vi "T7 Stream Read KAG-v2.vi"(0 "Connection ID In":refnum<k5>, 7 "Stream Configuration":T2={"Scan Rate (Hz)"=1000.0, "Samples Per Packet"=512, "Resolution Index"=0, "Buffer Size (bytes)"=32768, "NumScans"=1500, "Read Timeout (ms)"=5000, "Scan Table"=[{"Channel"=0, "BipGain"=0, "Input Config"="Single-Ended"}, {"Channel"=1, "BipGain"=0, "Input Config"="Single-Ended"}, {"Channel"=2, "BipGain"=0, "Input Config"="Single-Ended"}, {"Channel"=3, "BipGain"=0, "Input Config"="Single-Ended"}]} {"Samples Per Packet" max=512 step=1; "Buffer Size (bytes)" max=32768 step=1; "Resolution Index" max=8 step=1; "Scan Rate (Hz)" max=100000; "Scan Table"."BipGain" items=["x1", "x10", "x100", "x1000"]; "Scan Table"."Channel" step=1}, 9 "Secondary Stream Configurations":T1={"Settling Delay (*5 us)"=0.0, "Clock Source"=0, "Auto Target"=1} {"Auto Target" max=255 step=1; "Clock Source" max=2 step=2; "Settling Delay (*5 us)" min=0 max=5000 step=1}, 11 "error in":errorcluster) -> (6 "Read Array":u8[](array[numeric]) format="%.0x", 8 "TCP Data":string, 15 "error out":errorcluster)   [LabVIEW 2022 SP3]
doc: "Read Stream Data at Ethernet Socket 702."
uses:
  T7 Stream Config KAG.ctl
  T7 Secondary Configs KAG.ctl
  T7 Stream Globals KAG.vi
panel:
  in  "Tab Control":enum32{"TCP Read Data"}(tab)
  out "# of bytes received":i32
  out "# Bytes to Read":i32
  out "Scan Interval(s)":dbl
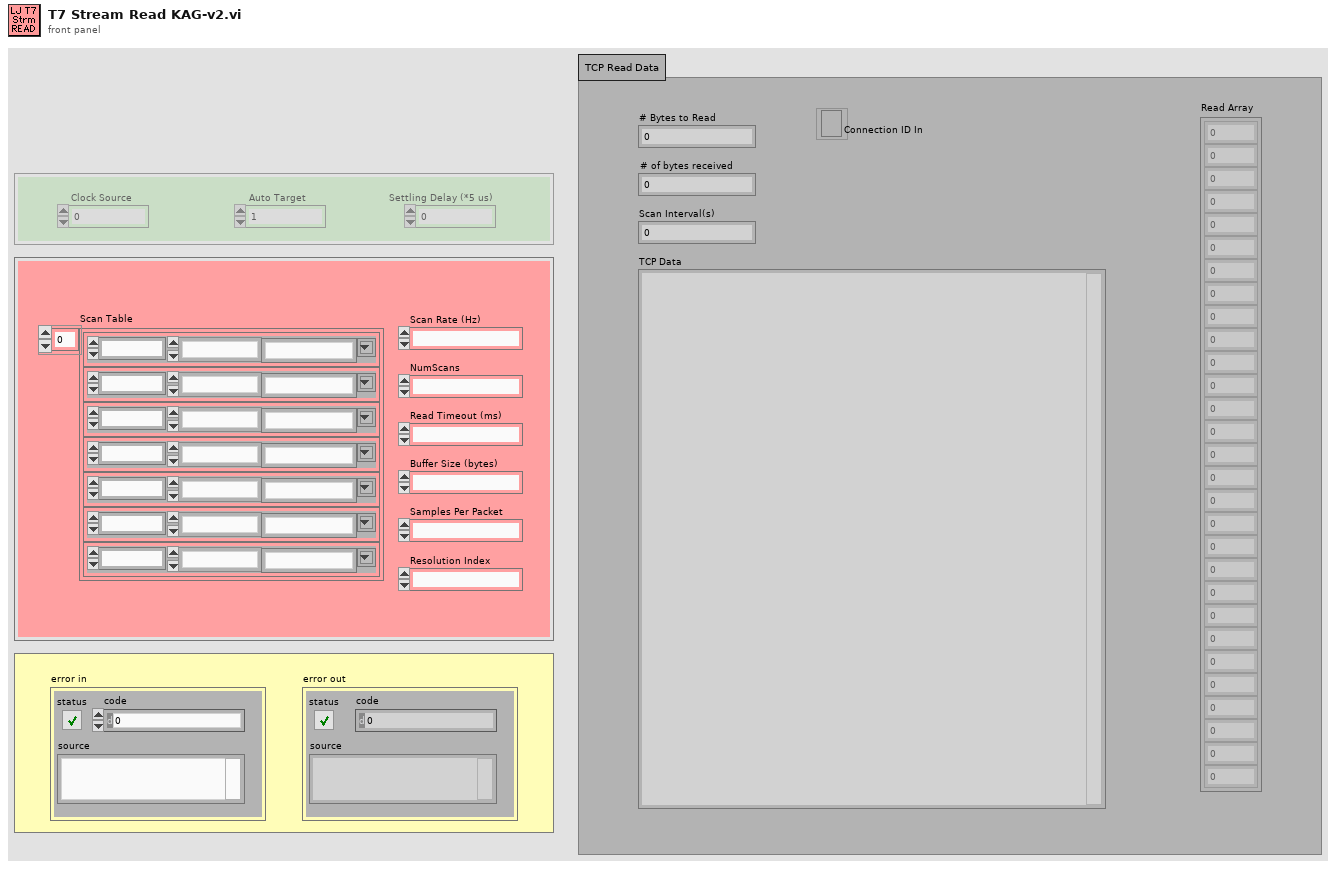
[diagram p1: front panel]
types:
  T1 = typedef "T7 Secondary Configs KAG.ctl" = cluster{"Settling Delay (*5 us)":sgl, "Clock Source":u32, "Auto Target":u32}
  T2 = typedef "T7 Stream Config KAG.ctl" = cluster{"Scan Rate (Hz)":sgl, "Samples Per Packet":u32, "Resolution Index":u32, "Buffer Size (bytes)":u32, "NumScans":u32, "Read Timeout (ms)":u32, "Scan Table":cluster{"Channel":u32, "BipGain":u32, "Input Config":string}[]}
  T3 = cluster{"Channel":u32, "BipGain":u32, "Input Config":string}[]
  T4 = typedef "T7 IP Config KAG.ctl" = cluster{"Connection ID In":refnum<k5>, "Connection ID Out":refnum<k5>, "Device IP":string, "Port":i32}
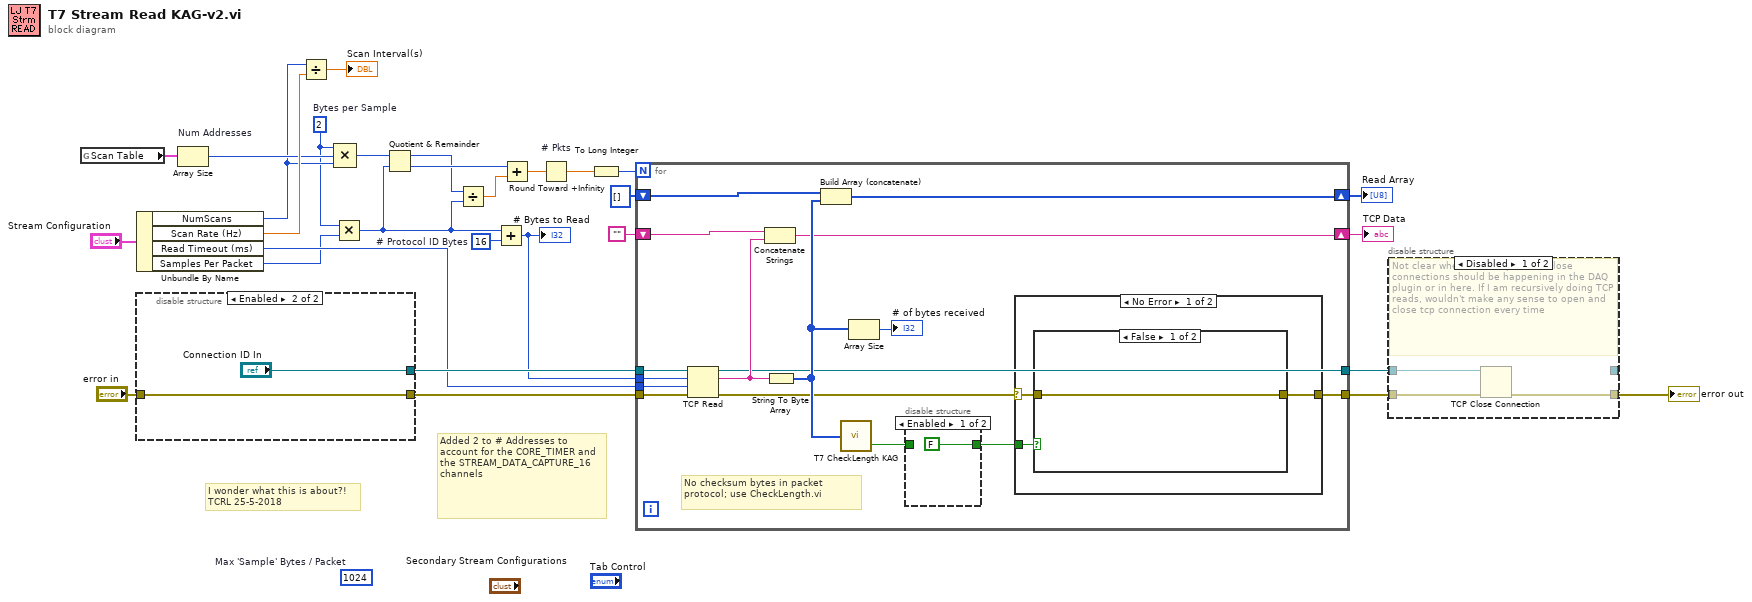
[diagram p0: block diagram]
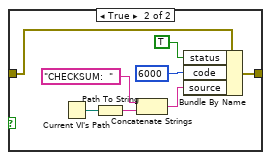
[diagram p4: hidden frame]
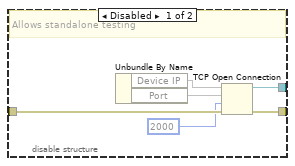
[diagram p6: hidden frame]
diagram:
  w2 = u32 16  # # Protocol ID Bytes
  (unwired) 1024  # Max 'Sample' Bytes / Packet
  w8 = 2  # Bytes per Sample
  # "I wonder what this is about?!\nTCRL 25-5-2018"
  # "Added 2 to # Addresses to account for the CORE_TIMER and the STREAM_DATA_CAPTURE_16 channels"
  n1 = global read "T7 Stream Globals KAG.vi" "Scan Table"() -> (w23:T3)
  n2 = Unbundle By Name("Stream Configuration") -> ("NumScans"=w18:u32, "Scan Rate (Hz)"=w20:sgl, "Read Timeout (ms)"=w21:u32, "Samples Per Packet"=w9:u32)
  n3 = disable-structure shown="Enabled" {
    disable-tunnel: "error in" -> [w36 w38]
    disable-tunnel: [w35 w38] -> w27
    disable-tunnel: [w34 "Connection ID In"] -> w26
    frame Disabled {
      # "Allows standalone testing"
      n4 = Unbundle By Name() -> (w33:T4, "Device IP"=w32, "Port"=w31)
      n5 = TCP Open Connection(address=w32, remote port or service name=w31, timeout ms (60000)=2000, error in (no error)=w36) -> (connection ID=w34:refnum<k5>, error out=w35:errorcluster)  [unwired: 1 out]
    }
    frame Enabled {
    }
  }
  n6 = Array Size "Num Addresses"(array=w23) -> (size(s)=w19:i32)
  n7 = Divide(x=w18, y=w20) -> (x/y=→"Scan Interval(s)":sgl)
  n8 = Compound Arithmetic op=MULTIPLY(w8, w19, w18) -> (w17:u32)
  n9 = Multiply(x=w8, y=w9) -> (x*y=w7:u32)
  n10 = Quotient & Remainder(x=w17, y=w7) -> (x-y*floor(x/y)=w6:u32, floor(x/y)=w15:u32)
  n11 = Divide(x=w6, y=w7) -> (x/y=w16:dbl)
  n12 = Add(x=w7, y=w2) -> (x+y=w1:u32)
  "# Bytes to Read" <- w1
  n13 = Add(x=w15, y=w16) -> (x+y=w14:dbl)
  n14 = Round Toward +Infinity "# Pkts"(x=w14) -> (ceil(x): smallest int >= x=w13:dbl)
  n15 = To Long Integer(number=w13) -> (32bit integer=w12:i32)
  n16 = for {
    N: w12 -> [_]
    tunnel: w27 -> [w53]
    tunnel: w26 -> [w52]
    tunnel: w21 -> [w49]
    shift-right: [w47] -> w25
    shift-left: u8[] [] ("unsigned byte array") -> [w46]
    shift-right: [w43] -> w29
    shift-left: "" -> [w45]
    tunnel: [w42] -> w4
    tunnel: [w41] -> w5
    tunnel: w1 -> [w39]
    # "No checksum bytes in packet protocol; use CheckLength.vi"
    n17 = TCP Read(connection ID=w52, bytes to read=w39, error in (no error)=w53, 9:w49) -> (connection ID out=w41:refnum<k5>, data out=w44:string, error out=w40:errorcluster)  [unwired: 1 out]
    n18 = Concatenate Strings(w45, w44) -> (w43:string)
    n19 = String To Byte Array(string=w44) -> (unsigned byte array=w48:u8[])
    n20 = Build Array (concatenate)(w46, w48) -> (w47:u8[])
    n21 = call "T7 CheckLength KAG.vi"("Array"=w48) -> ("CheckLength Error"=w50:bool)  [unwired: 1 out]
    n22 = Array Size(array=w48) -> (size(s)=→"# of bytes received":i32)
    n23 = disable-structure shown="Enabled" {
      disable-tunnel: [FALSE w56] -> w51
      disable-tunnel: w50 -> [_ w56]
      frame Enabled {
      }
      frame Disabled {
      }
    }
    n24 = case shown="No Error" w40 {
      selector: w40 -> [w59 w69]
      tunnel: [w58 w69] -> w42
      tunnel: w51 -> [w57 _]
      frame No Error {
        n25 = case shown="False" w57 {
          tunnel: w59 -> [w60 w68]
          tunnel: [w60 w67] -> w58
          frame False {
          }
          frame True {
            n26 = Current VI's Path() -> (path=w65:path)
            n27 = Path To String(path=w65) -> (string=w63:string)
            n28 = Concatenate Strings("CHECKSUM:  " ("Substring"), w63) -> (w62:string)
            n29 = Bundle By Name(cluster=w68, "status"=TRUE, "code"=u32 6000 ("y"), "source"=w62) -> (w67:errorcluster)
          }
        }
      }
      frame Error {
      }
    }
  }
  "Read Array" <- w25
  "TCP Data" <- w29
  n30 = disable-structure shown="Disabled" {
    disable-tunnel: w5 -> [w72 w74]
    disable-tunnel: w4 -> [w71 w73]
    disable-tunnel: [_ w74] -> _
    disable-tunnel: [w70 w73] -> w3
    frame Disabled {
      # "Not clear whether the open and close connections should be happening in the DAQ plugin or in here. If I am recursively doing TCP reads, wouldn't make any sense to open and close tcp connection every time"
      n31 = TCP Close Connection(connection ID=w72, error in (no error)=w71) -> (error out=w70:errorcluster)  [unwired: 1 in, 1 out]
    }
    frame Enabled {
    }
  }
  "error out" <- w3
